vi "Teleop.vi"(10 "Match Info":T1={"Autonomous Elapsed Seconds"=0.0, "TeleOp Elapsed Seconds"=0.0, "Disabled Elapsed Seconds"=0.0, "Visited Autonomous"=FALSE, "Visited TeleOp"=FALSE, "Visited Disabled"=FALSE, "Autonomous Settings"={"Autonomous Style"=enum."Independent", "VI Refnum"=refnum}}, 11 "Call Context":T2) -> ()   [LabVIEW 2017]
doc: "This VI is called for each enabled TeleOp packet received from the DS. It is typically used to read from joysticks and other inputs and update I/O or setpoints for timed control loops. It should complete and return within 20 milliseconds or risk missing DS packets."
uses:
  <vilib>/Rock Robotics/WPI/DriverStation/WPI_DriverStationDerivedRobotMode.ctl
  <vilib>/Rock Robotics/WPI/DriverStation/WPI_DriverStationMatch Info.ctl
  <vilib>/Rock Robotics/WPI/Utilities/WPI_GetSetVariantRefNum.vi
  <vilib>/Rock Robotics/Network Tables/NT Write Boolean Array.vi
  <vilib>/Rock Robotics/Network Tables/NT Write Numeric Array.vi
panel:
  out "f 2":dbl
  out "f":dbl
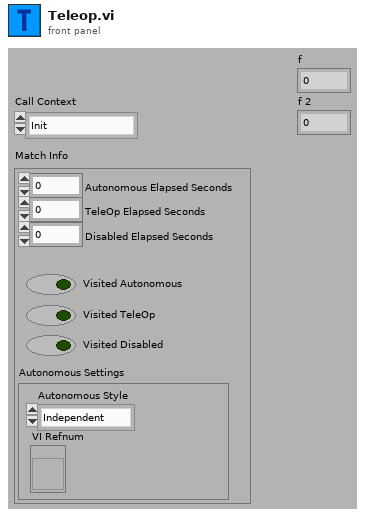
[diagram p1: front panel]
types:
  T1 = typedef "WPI_DriverStationMatch Info.ctl" = cluster{"Autonomous Elapsed Seconds":dbl, "TeleOp Elapsed Seconds":dbl, "Disabled Elapsed Seconds":dbl, "Visited Autonomous":bool, "Visited TeleOp":bool, "Visited Disabled":bool, "Autonomous Settings":cluster{"Autonomous Style":enum16{"Iterative", "Independent"}, "VI Refnum":refnum<vi>}}
  T2 = typedef "WPI_DriverStationDerivedRobotMode.ctl" = enum16{"Init", "Execute", "Stop"}
  T3 = typedef "WPI_JoystickDevRef.ctl" = cluster{"Device":T4}
  T4 = typedef "WPI_JoystickDeviceEnum.ctl" = enum16{"USB 0", "USB 1", "USB 2", "USB 3", "USB 4", "USB 5"}
  T5 = typedef "Command Status Info.ctl" = cluster{"Name":string, "Status":T6, "notifier out":T7}
  T6 = typedef "Completion Status.ctl" = enum16{"Successful", "Aborted", "Incomplete"}
  T7 = typedef "Completion Notifier.ctl" = refnum<notifier>
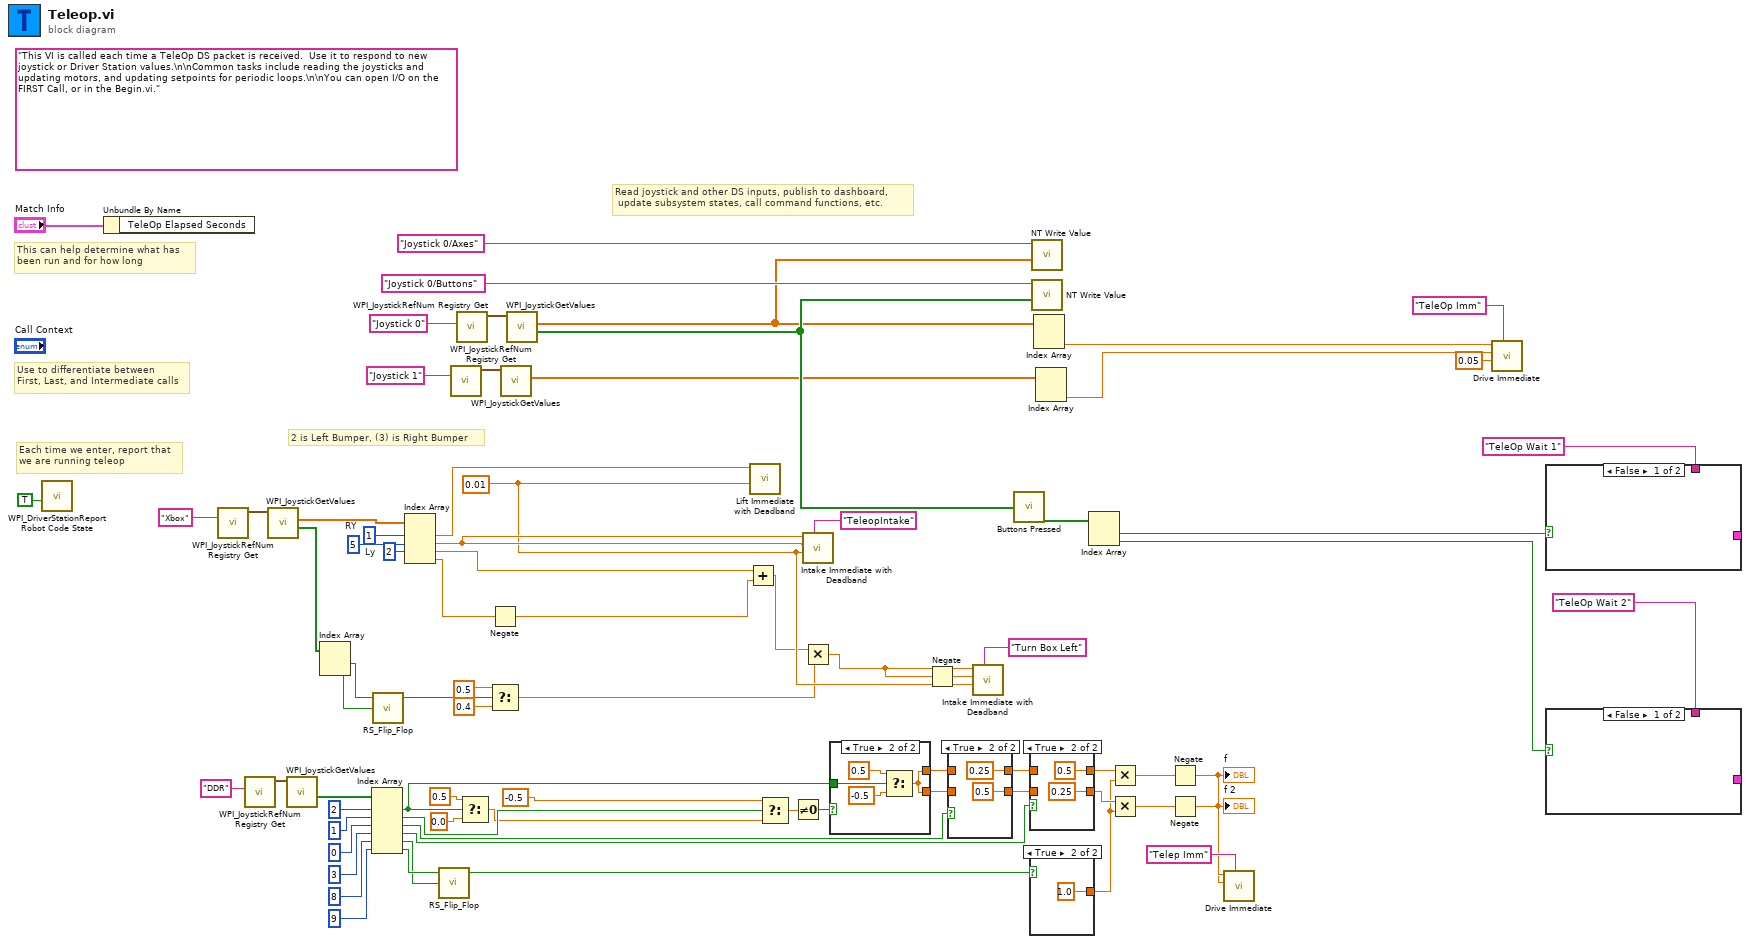
[diagram p0: block diagram]
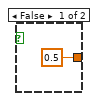
[diagram p2: hidden frame]
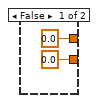
[diagram p5: hidden frame]
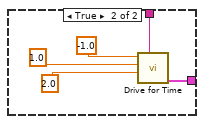
[diagram p6: hidden frame]
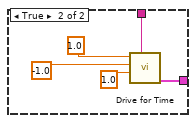
[diagram p7: hidden frame]
diagram:
  w55 = 5  # RY
  w56 = 1  # Ly
  w12 = 0.01 ("Deadband Value")
  (unwired) "This VI is called each time a TeleOp DS packet is received.  Use it to respond to new joystick or Driver Station values.\n\nCommon tasks include reading the joysticks and updating motors, and updating setpoints for periodic loops.\n\nYou can open I/O on the FIRST Call, or in the Begin.vi."
  # "2 is Left Bumper, (3) is Right Bumper"
  # "Read joystick and other DS inputs, publish to dashboard,\n update subsystem states, call command functions, etc."
  # "Each time we enter, report that\nwe are running teleop"
  # "Use to differentiate between\nFirst, Last, and Intermediate calls"
  # "This can help determine what has\nbeen run and for how long"
  n1 = call <vilib>:"WPI_DriverStationReport Robot Code State.vi"("TeleOp"=TRUE ("Autonomous")) -> ()  [unwired: 10 in, 1 out]
  n2 = Unbundle By Name("Match Info") -> ()  [unwired: 1 out]
  n3 = call <vilib>:"WPI_JoystickRefNum Registry Get.vi"("refnum name"="Xbox") -> ("JoystickDevRef"=w59:T3)  [unwired: 1 in, 9 out]
  n4 = call <vilib>:"WPI_JoystickRefNum Registry Get.vi"("refnum name"="DDR") -> ("JoystickDevRef"=w51:T3)  [unwired: 1 in, 9 out]
  n5 = call <vilib>:"WPI_JoystickGetValues.vi"("JoystickDevRef"=w59) -> ("Buttons"=w8:bool[], "Axes"=w58:dbl[])  [unwired: 6 in, 3 out]
  n6 = call <vilib>:"WPI_JoystickGetValues.vi"("JoystickDevRef"=w51) -> ("Buttons"=w50:bool[])  [unwired: 6 in, 4 out]
  n7 = Index Array(array=w8) -> (element #1=w7:bool, element #2=w6:bool)  [unwired: 2 in]
  n8 = Index Array(array=w50, index #1=2 ("index"), index #2=1 ("index"), index #3=0 ("index"), index #4=3 ("index"), index #5=8 ("index"), index #6=9 ("index")) -> (element #1=w31:bool, element #2=w45:bool, element #3=w35:bool, element #4=w32:bool, element #5=w27:bool, element #6=w28:bool)
  n9 = call "RS_Flip_Flop.vi"("Set"=w6, "Reset"=w7) -> ("Q"=w3:bool)  [unwired: 1 in, 2 out]
  n10 = Index Array(array=w58, index #1=w56, index #2=w55, index #3=2 ("index")) -> (element #1=w54:dbl, element #2=w15:dbl, element #3=w4:dbl, element #4=w11:dbl)  [unwired: 1 in]
  n11 = call "RS_Flip_Flop.vi"("Set"=w27, "Reset"=w28) -> ("Q"=w26:bool)  [unwired: 1 in, 2 out]
  n12 = call <vilib>:"WPI_JoystickRefNum Registry Get.vi"("refnum name"="Joystick 1") -> ("JoystickDevRef"=w64:T3)  [unwired: 1 in, 9 out]
  n13 = call <vilib>:"WPI_JoystickRefNum Registry Get.vi"("refnum name"="Joystick 0") -> ("JoystickDevRef"=w75:T3)  [unwired: 1 in, 9 out]
  n14 = Select(t=0.5, s=w31, f=0.0) -> (s? t:f=w42:dbl)
  n15 = Negate(x=w11) -> (-x=w10:dbl)
  n16 = Select(t=0.5 ("y"), s=w3, f=0.4) -> (s? t:f=w5:dbl)
  n17 = call <vilib>:"WPI_JoystickGetValues.vi"("JoystickDevRef"=w64) -> ("Axes"=w63:dbl[])  [unwired: 6 in, 4 out]
  n18 = call <vilib>:"WPI_JoystickGetValues.vi"("JoystickDevRef"=w75) -> ("Buttons"=w68:bool[], "Axes"=w67:dbl[])  [unwired: 6 in, 3 out]
  n19 = Add(x=w4, y=w10) -> (x+y=w9:dbl)
  n20 = call "Lift Immediate with Deadband.vi"("Deadband Value"=w12, "Setpoint"=w54) -> ()  [unwired: 9 in, 1 out]
  n21 = Select(t=-0.5, s=w45, f=w42) -> (s? t:f=w38:dbl)
  n22 = Not Equal To 0?(x=w38) -> (x != 0?=w39:bool)
  n23 = call "Intake Immediate with Deadband.vi"("Left Setpoint"=w15, "Right Setpoint"=w15, "Deadband Value"=w12, "Description"="TeleopIntake") -> ()  [unwired: 6 in, 1 out]
  n24 = Multiply(x=w9, y=w5) -> (x*y=w14:dbl)
  n25 = case shown="True" w39 {
    tunnel: [0.0 w82] -> w36
    tunnel: [0.0 w82] -> w37
    tunnel: w31 -> [_ w81]
    frame False {
    }
    frame True {
      n26 = Select(t=0.5, s=w81, f=-0.5) -> (s? t:f=w82:dbl)
    }
  }
  n27 = Negate(x=w14) -> (-x=w16:dbl)
  n28 = case shown="True" w35 {
    tunnel: w37 -> [w86 _]
    tunnel: w36 -> [w85 _]
    tunnel: [w86 0.25 ("f")] -> w34
    tunnel: [w85 0.5 ("f")] -> w33
    frame False {
    }
    frame True {
    }
  }
  n29 = call "Intake Immediate with Deadband.vi"("Left Setpoint"=w14, "Right Setpoint"=w16, "Deadband Value"=w12, "Description"="Turn Box Left") -> ()  [unwired: 6 in, 1 out]
  n30 = call "Buttons Pressed.vi"("Button Values"=w68) -> ("Button Presses"=w72:bool[])
  n31 = case shown="True" w32 {
    tunnel: w34 -> [w90 _]
    tunnel: w33 -> [w89 _]
    tunnel: [w90 0.5 ("f")] -> w25
    tunnel: [w89 0.25 ("f")] -> w24
    frame False {
    }
    frame True {
    }
  }
  n32 = case shown="True" w26 {
    tunnel: [0.5 1.0] -> w23
    frame False {
    }
    frame True {
    }
  }
  n33 = call-poly <vilib>:"NT Write Value.vi"("Numeric Array"=w67, "Name"="Joystick 0/Axes") -> ()  [unwired: 9 in, 1 out]
  n34 = call-poly <vilib>:"NT Write Value.vi"("Boolean Array"=w68, "Name"="Joystick 0/Buttons") -> ()  [unwired: 9 in, 1 out]
  n35 = Index Array(array=w67) -> (element #2=w61:dbl)  [unwired: 2 in, 1 out]
  n36 = Index Array(array=w63) -> (element #2=w62:dbl)  [unwired: 2 in, 1 out]
  n37 = Index Array(array=w72) -> (element #1=w71:bool, element #2=w70:bool)  [unwired: 2 in]
  n38 = Multiply(x=w25, y=w23) -> (x*y=w21:dbl)
  n39 = Multiply(x=w24, y=w23) -> (x*y=w20:dbl)
  n40 = Negate(x=w21) -> (-x=w22:dbl)
  "f" <- w22
  n41 = Negate(x=w20) -> (-x=w19:dbl)
  "f 2" <- w19
  n42 = call "Drive Immediate.vi"("Description"="Telep Imm", "Right Setpoint"=w19, "Left Setpoint"=w22) -> ()  [unwired: 8 in, 1 out]
  n43 = call "Drive Immediate.vi"("Description"="TeleOp Imm", "Deadband Value"=0.05, "Right Setpoint"=w62, "Left Setpoint"=w61) -> ()  [unwired: 7 in, 1 out]
  n44 = case shown="False" w71 {
    tunnel: [_ w98] -> _
    tunnel: "TeleOp Wait 1" ("Description") -> [_ w97]
    frame False {
    }
    frame True {
      n45 = call "Drive for Time.vi"("Description"=w97, "Seconds"=1.0, "Right Speed"=-1.0, "Left Speed"=1.0) -> ("Command Info Out"=w98:T5)  [unwired: 6 in, 1 out]
    }
  }
  n46 = case shown="False" w70 {
    tunnel: [_ w102] -> _
    tunnel: "TeleOp Wait 2" ("Description") -> [_ w101]
    frame False {
    }
    frame True {
      n47 = call "Drive for Time.vi"("Description"=w101, "Seconds"=2.0, "Right Speed"=1.0, "Left Speed"=-1.0) -> ("Command Info Out"=w102:T5)  [unwired: 6 in, 1 out]
    }
  }
